vi "Handling AO param.vi"(8 "error in (no error)":errorcluster, 9 "AO":dbl[](array[numeric]), 10 "AOP":dbl[][](array[numeric]), 11 "AOint_def":u16[][](array[numeric])) -> (0 "error":errorcluster, 3 "AOint":u16[][](array[numeric]))   [LabVIEW 2019, in "Inputs.lvlib"]
uses:
  Inputs.lvlib
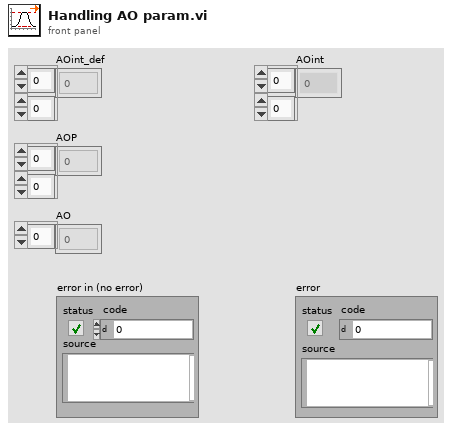
[diagram p1: front panel]
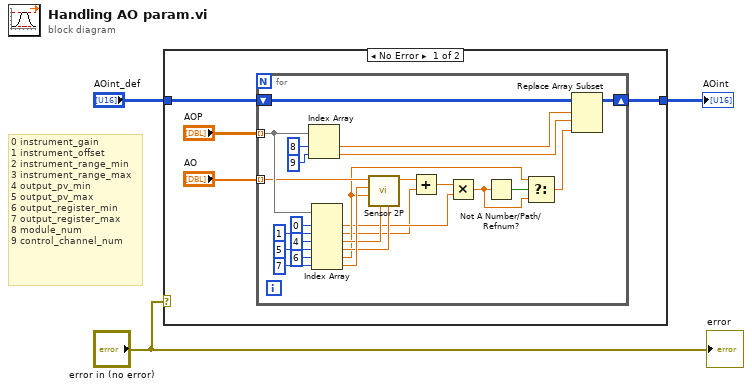
[diagram p0: block diagram]
diagram:
  # "0 instrument_gain\n1 instrument_offset\n2 instrument_range_min\n3 instrument_range_max\n4 output_pv_min\n5 output_pv_max\n6 output_register_min\n7 output_register_max\n8 module_num\n9 control_channel_num"
  n1 = case shown="No Error" "error in (no error)" {
    tunnel: "AOint_def" -> [w5 w33]
    tunnel: [w4 w33] -> w2
    frame No Error {
      n2 = for {
        tunnel: "AOP" -> [w25] mode=indexing
        shift-right: [w30] -> w4
        shift-left: w5 -> [w29]
        tunnel: "AO" -> [w20] mode=indexing
        n3 = Index Array(array=w25, index #1=8 ("index (row)"), index #2=9 ("index (row)")) -> (element #1=w16:dbl, element #2=w15:dbl)
        n4 = Index Array(array=w25, index #1=0 ("disabled index (col)"), index #2=1 ("disabled index (col)"), index #3=4 ("disabled index (col)"), index #4=5 ("disabled index (col)"), index #5=6 ("disabled index (col)"), index #6=7 ("disabled index (col)")) -> (element #1=w9:dbl, element #2=w8:dbl, element #3=w26:dbl, element #4=w27:dbl, element #5=w18:dbl, element #6=w28:dbl)
        n5 = call "Sensor 2P.vi"("Xmax"=w27, "Xmin"=w26, "Ymin"=w18, "Ymax"=w28, "X"=w20) -> ("Y"=w12:dbl)  [unwired: 6 in]
        n6 = Add(x=w12, y=w8) -> (x+y=w14:dbl)
        n7 = Multiply(x=w14, y=w9) -> (x*y=w13:dbl)
        n8 = Not A Number/Path/Refnum?(number/path/refnum=w13) -> (NaN/Path/Refnum?=w19:bool)
        n9 = Select(t=w18, s=w19, f=w13) -> (s? t:f=w17:dbl)
        n10 = Replace Array Subset(array=w29, new element=w17, index (row)=w16, index (col)=w15) -> (w30:u16[][])
      }
    }
    frame Error {
    }
  }
  "AOint" <- w2
  "error" <- "error in (no error)"
